vi "Sensor+Pump_Labview.vi"() -> ()   [LabVIEW 2020]
uses:
  <vilib>/Instr/_visa.llb/VISA Configure Serial Port (Instr).vi
panel:
  out "return count":u32
  out "concatenated string":string
  out "error out":errorcluster
  in  "Arduino COM Port":refnum<visa-resource-name>
  out "voltage soil":dbl
  in  "stop":bool
  out "Pump Command":string
  out "Pump Duration (s)":dbl
  out "Moisture Deficit (%)":dbl
  out "Humidity (%)":dbl
  out "Temperature (°C)":dbl
  out "Soil Moisture (%)":dbl
  in  "Maximum Pump Time (s)":dbl
  in  "K Value":dbl
  in  "Target Moisture (%)":dbl
  in  "Humidity High Voltage":dbl
  in  "Humidity Low Voltage":dbl
  in  "Vwet":dbl
  in  "Vdry":dbl
  in  "AM1001 Humidity Voltage":dbl
  in  "LM35 Temperature Voltage":dbl
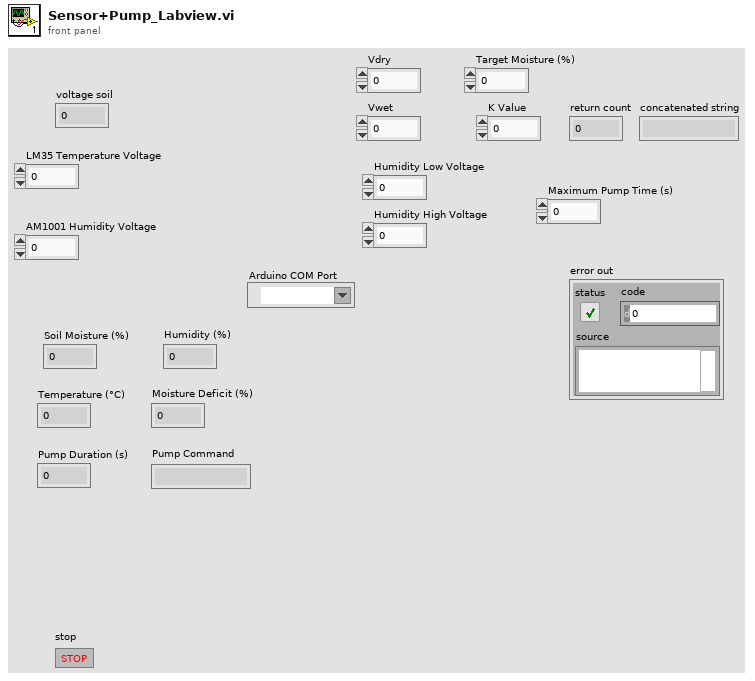
[diagram p1: front panel]
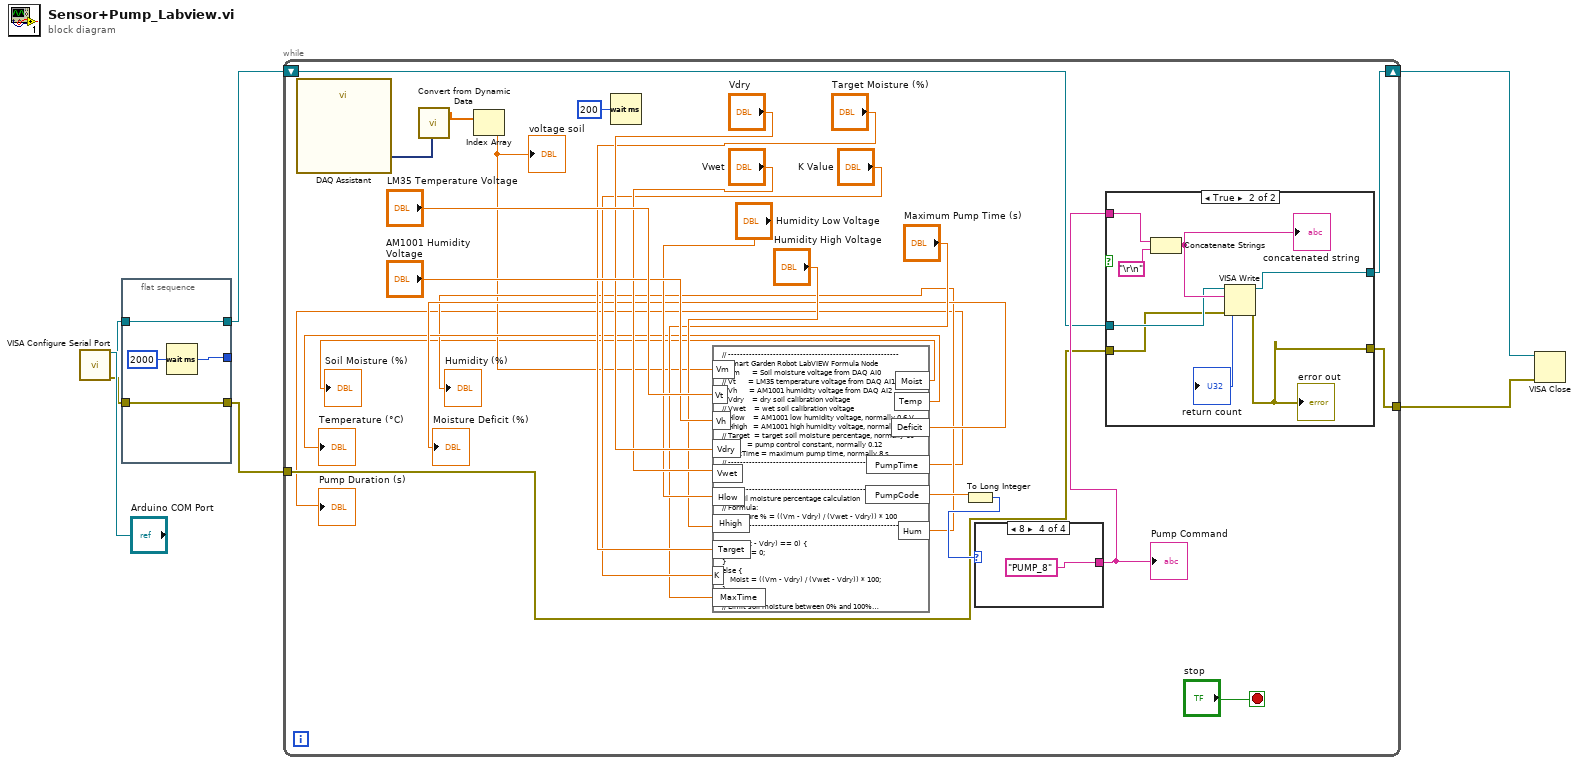
[diagram p0: block diagram]
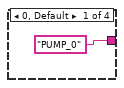
[diagram p3: hidden frame]
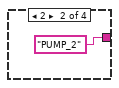
[diagram p4: hidden frame]
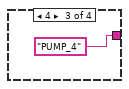
[diagram p5: hidden frame]
diagram:
  n1 = call-poly "VISA Configure Serial Port"("VISA resource name"="Arduino COM Port") -> ("VISA resource name out"=w6:refnum<visa-resource-name>, "error out"=w5:errorcluster)  [unwired: 13 in]
  n2 = flat-sequence {
    tunnel: [w11] -> _
    tunnel: [w9] -> w4
    tunnel: w6 -> [w9]
    tunnel: [w8] -> w3
    tunnel: w5 -> [w8]
    frame #0 {
      n3 = Wait (ms)(milliseconds to wait=u32 2000) -> (millisecond timer value=w11:u32)
    }
  }
  n4 = while {
    shift-right: [w16] -> w2
    shift-left: w4 -> [w17]
    tunnel: w3 -> [w15]
    tunnel: [w14] -> w1
    stop <- "stop" stop-if-true
    n5 = call "DAQ Assistant"() -> ("data"=w21:dynamicdata)  [unwired: 16 in, 3 out]
    n6 = call "Convert from Dynamic Data"("Dynamic Data Type"=w21) -> ("Array"=w20:dbl[])  [unwired: 3 in]
    n7 = Index Array(array=w20) -> (element=w19:dbl)  [unwired: 1 in]
    "voltage soil" <- w19
    n8 = Wait (ms)(milliseconds to wait=u32 200) -> ()  [unwired: 1 out]
    n9 = formula code="// ---------------------------------------------------------\n// Smart Garden Robot LabVIEW Formula Node\n// Vm      = Soil moisture voltage from DAQ AI0\n// Vt      = LM35 temperature voltage from DAQ AI1\n// Vh      = AM1001 humidity voltage from DAQ AI2\n// Vdry    = dry soil calibration voltage\n// Vwet    = wet soil calibration voltage\n// Hlow    = AM1001 low humidity voltage, normally 0.6 V\n// Hhigh   = AM1001 high humidity voltage, normally 2.7 V\n// Target  = target soil moisture percentage, normally 60\n// K       = pump control constant, normally 0.12\n// MaxTime = maximum pump time, normally 8 s\n// ---------------------------------------------------------\n\n\n// ---------------------------------------------------------\n// 1. Soil moisture percentage calculation\n// Formula:\n// Moisture % = ((Vm - Vdry) / (Vwet - Vdry)) * 100\n// ---------------------------------------------------------\n\nif ((Vwet - Vdry) == 0) {\n    Moist = 0;\n}\nelse {\n    Moist = ((Vm - Vdry) / (Vwet - Vdry)) * 100;\n}\n\n// Limit soil moisture between 0% and 100%\nif (Moist < 0) {\n    Moist = 0;\n}\n\nif (Moist > 100) {\n    Moist = 100;\n}\n\n\n// ---------------------------------------------------------\n// 2. LM35 temperature calculation\n// LM35 output = 10 mV per degree Celsius\n// Temperature = Vt / 0.01\n// ---------------------------------------------------------\n\nTemp = Vt / 0.01;\n\n\n// ---------------------------------------------------------\n// 3. AM1001 humidity calculation\n// Approximate AM1001 calibration:\n// 0.6 V = 20% RH\n// 2.7 V = 90% RH\n// Formula:\n// Humidity % = 20 + ((Vh - Hlow) / (Hhigh - Hlow)) * 70\n// ---------------------------------------------------------\n\nif ((Hhigh - Hlow) == 0) {\n    Hum = 0;\n}\nelse {\n    Hum = 20 + ((Vh - Hlow) / (Hhigh - Hlow)) * 70;\n}\n\n// Limit humidity between 0% and 100%\nif (Hum < 0) {\n    Hum = 0;\n}\n\nif (Hum > 100) {\n    Hum = 100;\n}\n\n\n// ---------------------------------------------------------\n// 4. Moisture deficit calculation\n// Deficit = Target moisture - Measured moisture\n// ---------------------------------------------------------\n\nDeficit = Target - Moist;\n\n\n// ---------------------------------------------------------\n// 5. Pump duration calculation\n// If moisture is enough, pump time = 0\n// If moisture is low, pump time = K * Deficit\n// Pump time is limited by MaxTime\n// ---------------------------------------------------------\n\nif (Deficit <= 0) {\n    PumpTime = 0;\n}\nelse {\n    PumpTime = K * Deficit;\n\n    if (PumpTime > MaxTime) {\n        PumpTime = MaxTime;\n    }\n}\n\n\n// ---------------------------------------------------------\n// 6. Pump command code\n// 0 = PUMP_0\n// 2 = PUMP_2\n// 4 = PUMP_4\n// 8 = PUMP_8\n// ---------------------------------------------------------\n\nif (PumpTime <= 0) {\n    PumpCode = 0;\n}\nelse if (PumpTime <= 2) {\n    PumpCode = 2;\n}\nelse if (PumpTime <= 4) {\n    PumpCode = 4;\n}\nelse {\n    PumpCode = 8;\n}"("Vm"=w19, "Vh"="AM1001 Humidity Voltage", "Vdry"="Vdry", "Vwet"="Vwet", "Hlow"="Humidity Low Voltage", "Hhigh"="Humidity High Voltage", "Target"="Target Moisture (%)", "K"="K Value", "MaxTime"="Maximum Pump Time (s)", "Vt"="LM35 Temperature Voltage") -> ("Moist"=→"Soil Moisture (%)":dbl, "Temp"=→"Temperature (°C)":dbl, "Deficit"=→"Moisture Deficit (%)":dbl, "PumpTime"=→"Pump Duration (s)":dbl, "PumpCode"=w25:dbl, "Hum"=→"Humidity (%)":dbl)
    n10 = To Long Integer(number=w25) -> (32bit integer=w24:i32)
    n11 = case shown="8" w24 {
      tunnel: ["PUMP_0" "PUMP_2" "PUMP_4" "PUMP_8"] -> w18
      frame 0, Default {
      }
      frame 2 {
      }
      frame 4 {
      }
      frame 8 {
      }
    }
    "Pump Command" <- w18
    n12 = case shown="True" {
      selector: _ -> [_ _]
      tunnel: w17 -> [w39 w45]
      tunnel: [w39 w40] -> w16
      tunnel: w15 -> [w38 w44]
      tunnel: [w38 w43] -> w14
      tunnel: w18 -> [_ w41]
      frame False {
      }
      frame True {
        n13 = Concatenate Strings(w41, "\r\n") -> (w46:string)
        "concatenated string" <- w46
        n14 = VISA Write(VISA resource name=w45, write buffer=w46, error in (no error)=w44) -> (VISA resource name out=w40:refnum<visa-resource-name>, return count=→"return count":u32, error out=w43:errorcluster)
        "error out" <- w43
      }
    }
  }
  n15 = VISA Close(VISA resource name=w2, error in (no error)=w1) -> ()  [unwired: 1 out]
